vi "servo act nation.vi"(8 "error in":errorcluster, 10 "servo act":T1) -> (0 "error out":errorcluster)   [LabVIEW 2019]
uses:
  ctl/servo act.ctl
  FPGA_subVIs/low level/Servo/Servo.enum.ctl
  FPGA_subVIs/my FPGA lib.lvlib
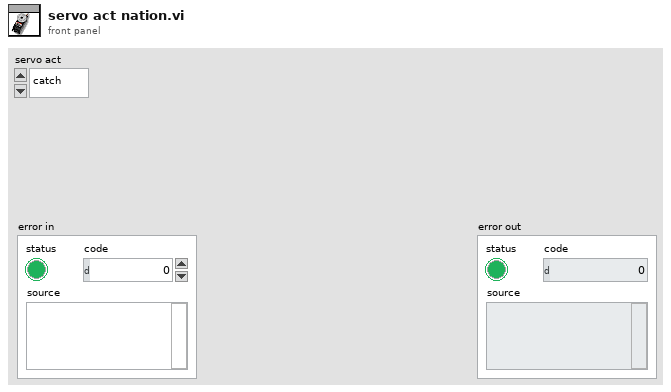
[diagram p1: front panel]
types:
  T1 = typedef "servo act.ctl" = enum16{"catch", "relax", "left idle", "center", "red relax", "left reg", "right reg"}
  T2 = typedef "my FPGA lib.lvlib/Servo.enum.ctl" = enum16{"Servo.1", "Servo.2", "Servo.3"}
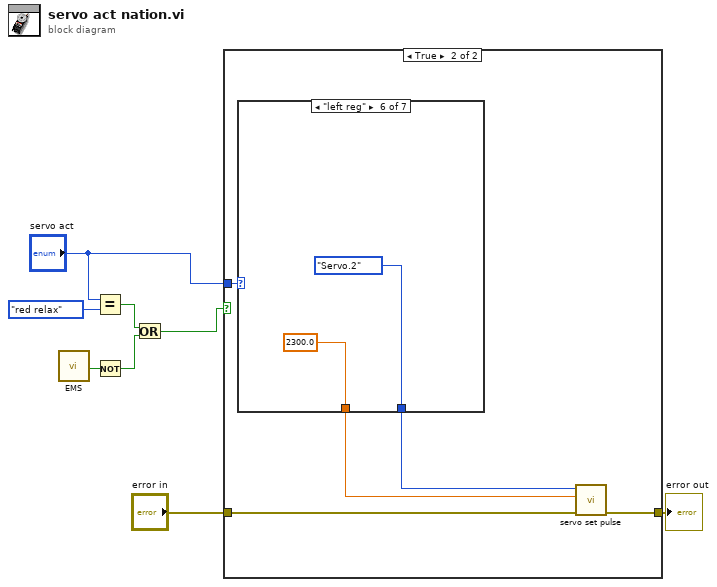
[diagram p0: block diagram]
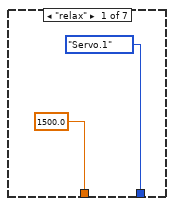
[diagram p3: hidden frame]
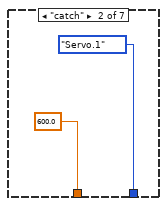
[diagram p4: hidden frame]
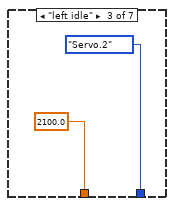
[diagram p5: hidden frame]
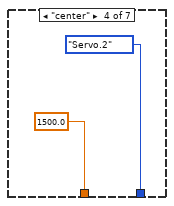
[diagram p6: hidden frame]
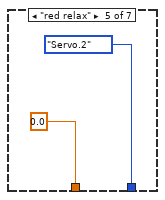
[diagram p7: hidden frame]
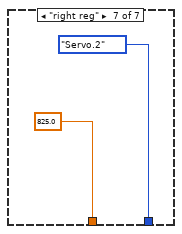
[diagram p8: hidden frame]
diagram:
  n1 = call "EMS.vi"() -> ("A/DIO4 (Pin 19)"=w4:bool)
  n2 = Equal?(x="servo act", y=servo_act."red relax") -> (x = y?=w3:bool)
  n3 = Not(x=w4) -> (.not. x?=w2:bool)
  n4 = Or(x=w3, y=w2) -> (x .or. y?=w1:bool)
  n5 = case shown="True" w1 {
    tunnel: "servo act" -> [_ w14]
    tunnel: "error in" -> [w9 w11]
    tunnel: [w9 w10] -> w7
    frame False {
    }
    frame True {
      n6 = case shown="\"left reg\"" w14 {
        tunnel: [Servo.enum."Servo.1" ("Enum") Servo.enum."Servo.1" ("Enum") Servo.enum."Servo.2" ("Enum") Servo.enum."Servo.2" ("Enum") Servo.enum."Servo.2" ("Enum") Servo.enum."Servo.2" ("Enum") Servo.enum."Servo.2" ("Enum")] -> w13
        tunnel: [1500.0 ("servo pulse(us)") 600.0 ("servo pulse(us)") 2100.0 ("servo pulse(us)") 1500.0 ("servo pulse(us)") 0.0 ("servo pulse(us)") 2300.0 ("servo pulse(us)") 825.0 ("servo pulse(us)")] -> w12
        frame "relax" {
        }
        frame "catch" {
        }
        frame "left idle" {
        }
        frame "center" {
        }
        frame "red relax" {
        }
        frame "left reg" {
        }
        frame "right reg" {
        }
      }
      n7 = call "servo set pulse.vi"("error in"=w11, "servo pulse(us)"=w12, "Enum"=w13) -> ("error out"=w10:errorcluster)  [unwired: 8 in]
    }
  }
  "error out" <- w7
